vi "extract info from binary file.vi"(8 "error in (no error)":errorcluster, 11 "Tomo in":refnum<class "Tomo.lvclass">) -> (0 "error out":errorcluster, 3 "Tomo out":refnum<class "Tomo.lvclass">)   [LabVIEW 2012, in "Tomo.lvclass"]
uses:
  Tomo.lvclass
  Tomo.lvclass/Tomo.ctl
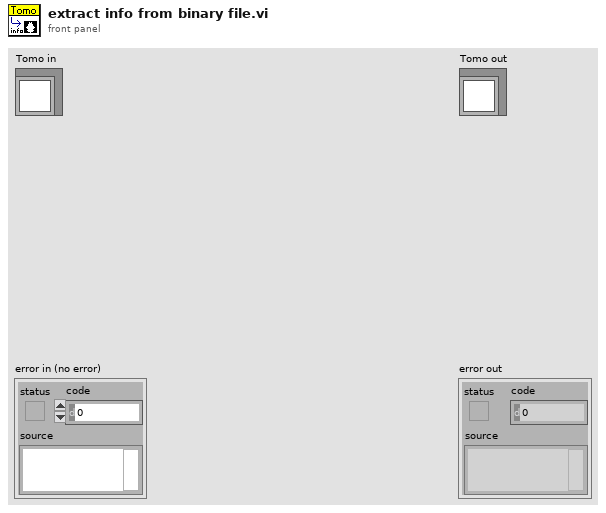
[diagram p1: front panel]
types:
  T1 = typedef "IMAQ Image.ctl" = refnum<image>
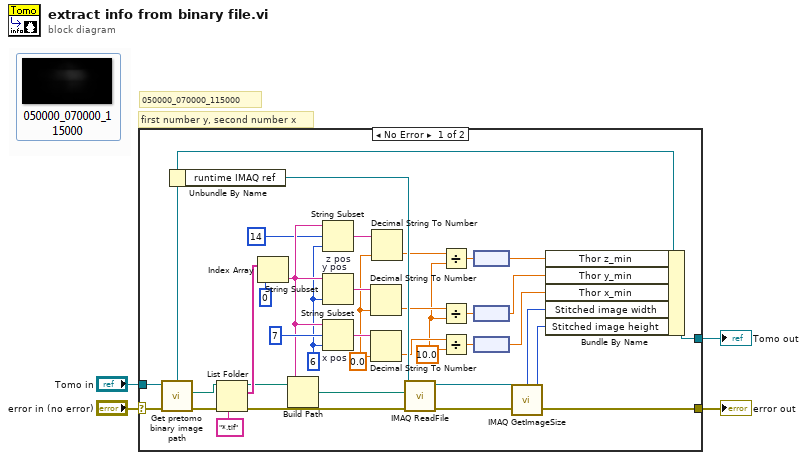
[diagram p0: block diagram]
diagram:
  # "first number y, second number x"
  # "050000_070000_115000"
  n1 = case shown="No Error" "error in (no error)" {
    selector: "error in (no error)" -> [w40 w42]
    tunnel: [w27 w42] -> w3
    tunnel: [w25 w41] -> w1
    tunnel: "Tomo in" -> [w30 w41]
    frame No Error {
      w7 = 10.0 ("y")
      w10 = 0.0
      w13 = 6 ("length (rest)")
      n2 = call-dynamic "Get pretomo binary image path.vi"("error in (no error)"=w40, "Tomo in"=w30) -> ("error out"=w39:errorcluster, "pretomo binary path"=w38:path, "Tomo out"=w26:refnum<class "Tomo.lvclass">)  [unwired: 6 in, 1 out]
      n3 = Unbundle By Name(w26) -> ("runtime IMAQ ref"=w31:T1)
      n4 = List Folder(path=w38, pattern="*.tif", error in=w39) -> (path out=w34:path, filenames=w36:string[], error out=w33:errorcluster)  [unwired: 1 in, 1 out]
      n5 = Index Array(array=w36, index=0) -> (element=w14:string)
      n6 = Build Path(base path=w34, name or relative path=w14) -> (appended path=w32:path)
      n7 = String Subset "z pos"(string=w14, offset (0)=14, length (rest)=w13) -> (substring=w11:string)
      n8 = String Subset "y pos"(string=w14, length (rest)=w13) -> (substring=w22:string)  [unwired: 1 in]
      n9 = String Subset "x pos"(string=w14, offset (0)=7, length (rest)=w13) -> (substring=w21:string)
      n10 = Decimal String To Number(string=w22, default (0L)=w10) -> (number=w9:dbl)  [unwired: 1 in, 1 out]
      n11 = Decimal String To Number(string=w21, default (0L)=w10) -> (number=w17:dbl)  [unwired: 1 in, 1 out]
      n12 = Decimal String To Number(string=w11, default (0L)=w10) -> (number=w8:dbl)  [unwired: 1 in, 1 out]
      n13 = call "IMAQ ReadFile"("File Path"=w32, "error in (no error)"=w33, "Image"=w31) -> ("error out"=w28:errorcluster, "Image Out"=w29:T1)  [unwired: 4 in, 3 out]
      n14 = Divide(x=w8, y=w7) -> (x/y=w6:dbl)
      n15 = Divide(x=w9, y=w7) -> (x/y=w15:dbl)
      n16 = Divide(x=w17, y=w7) -> (x/y=w16:dbl)
      n17 = node(w6) -> (w5:dbl[unit])
      n18 = node(w15) -> (w20:dbl[unit])
      n19 = node(w16) -> (w19:dbl[unit])
      n20 = call "IMAQ GetImageSize"("Image"=w29, "error in (no error)"=w28) -> ("Y Resolution"=w23:i32, "X Resolution"=w24:i32, "error out"=w27:errorcluster)  [unwired: 2 in]
      n21 = Bundle By Name(cluster=w26, "Thor z_min"=w5, "Thor y_min"=w20, "Thor x_min"=w19, "Stitched image width"=w24, "Stitched image height"=w23) -> (w25:refnum<class "Tomo.lvclass">)
    }
    frame Error {
    }
  }
  "error out" <- w3
  "Tomo out" <- w1
